vi "Dispose.vi"(0 "object in":refnum<class "XmlLogger.lvclass">, 5 "error in (no error)":errorcluster) -> (14 "object out":refnum<class "XmlLogger.lvclass">, 19 "error out":errorcluster)   [LabVIEW 2014, in "XmlLogger.lvclass"]
uses:
  XmlLogger.lvclass
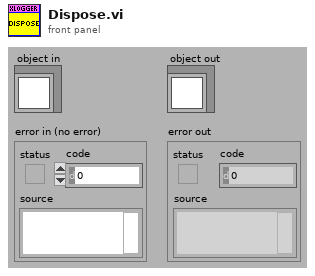
[diagram p1: front panel]
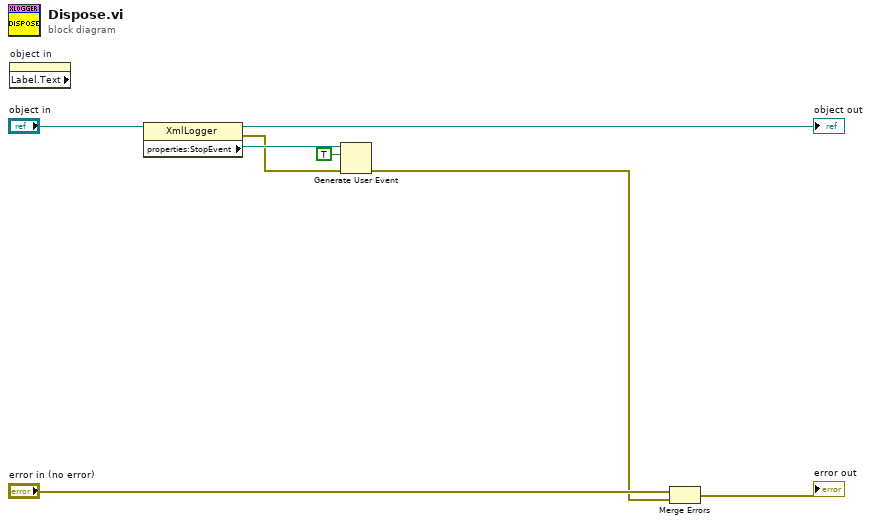
[diagram p0: block diagram]
diagram:
  n1 = property on="object in" class="LVClassControl (strict)" props=["Label", "Text"]() -> ()  [unwired: 2 in, 3 out]
  n2 = property class="XmlLogger"(reference="object in") -> (reference out=→"object out":refnum<class "XmlLogger.lvclass">, error out=w1:errorcluster, "properties:StopEvent"=w6:refnum<user-event>)  [unwired: 1 in]
  n3 = Generate User Event(user event=w6, event data cluster=TRUE ("event data"), error in=w1) -> (error out=w2:errorcluster)  [unwired: 1 in, 1 out]
  n4 = Merge Errors("error in (no error)", w2) -> (→"error out":errorcluster)
